vi "HEWH Draw Start GEA3 Commands.vi"(5 "Draw Station":string, 7 "GEA3?":bool, 8 "error in (no error)":errorcluster, 9 "Draw Parameters Seq":T1 {"Station D"."Time" format="%<%H:%M:%S>t"; "Station C"."Time" format="%<%H:%M:%S>t"; "Station B"."Time" format="%<%H:%M:%S>t"; "Station A"."Time" format="%<%H:%M:%S>t"}, 11 "GEA3 Reference Out":refnum<k24>) -> (0 "error out":errorcluster, 3 "GEA2 Reference Out":refnum<k24>)   [LabVIEW 2019]
uses:
  Type Definitions/HEWH Draw Parameters.ctl
  Type Definitions/PRAT Test.ctl
  Utility/Save File/File Setup (Public)/Type Definition/Save File HEWH Heating Control Mode.ctl
  Draw Water Specific/Type Definitions/Terminate Draw Conditions.ctl
  Type Definitions/HEWH Start Conditions.ctl
  Draw Water Specific/Type Definitions/Check Special Condtions.ctl
  Draw Water Specific/Type Definitions/HEWH Special Condition Check.ctl
  Type Definitions/HEWH Draw Flag ENUM.ctl
  C:/TechnologyLab/NI-2010/Drivers/GEA3 Toolkit/GEA3 DLL Source/GeaCommunication.dll
  Drivers/GEA3 Toolkit/GEA3 DLL Source/GeaCommunication.dll
  Drivers/GEA3 Toolkit/LabVIEW GEA3 Rev2 API Toolkit LV2016/type defs/ERD Write Data In.ctl
  Drivers/GEA3 Toolkit/LabVIEW GEA3 Rev2 API Toolkit LV2016/type defs/Data Type.ctl
  Utility/Save File/File Setup.lvlib
  Drivers/GEA3 Toolkit/LabVIEW GEA3 Rev2 API Toolkit LV2016/library/GEA2_Toolkit.lvlib
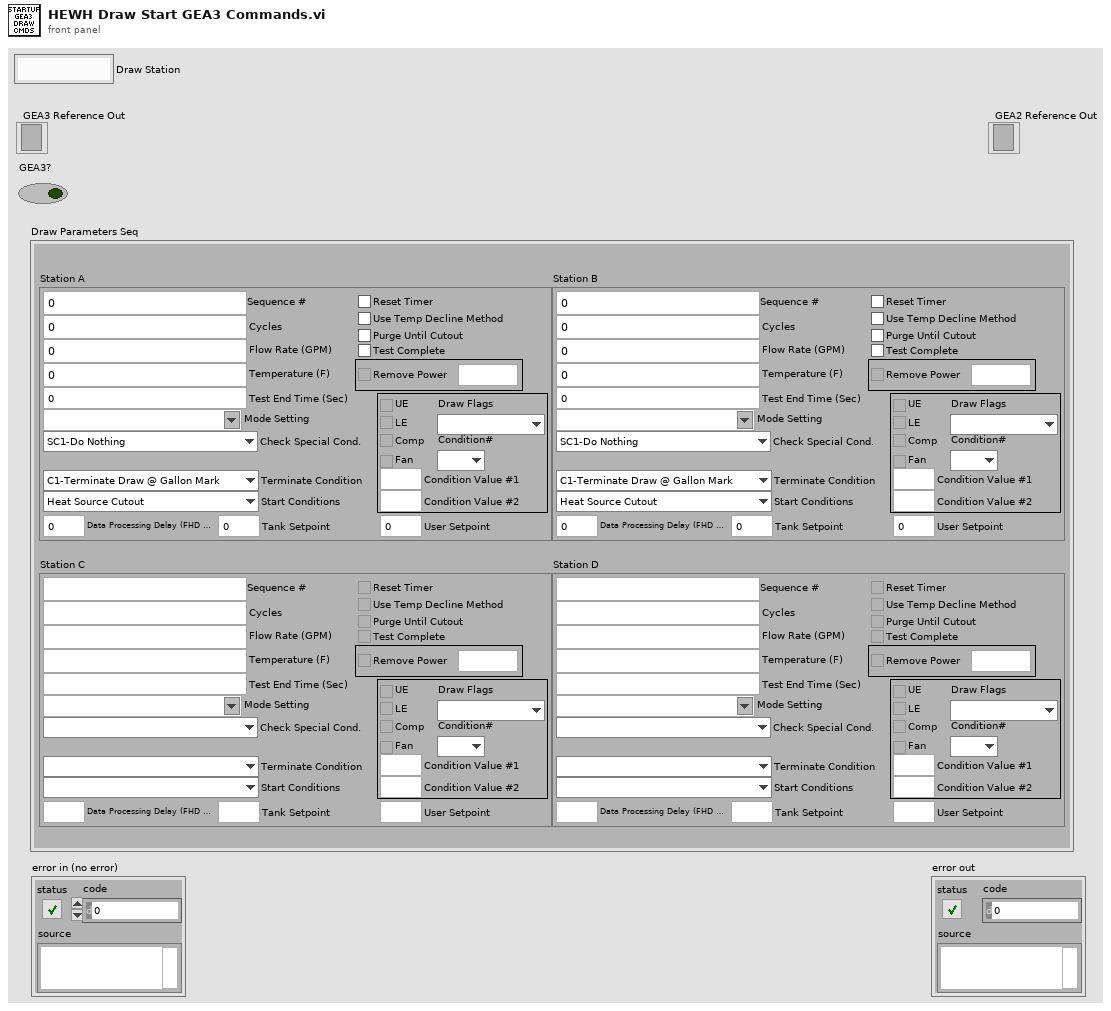
[diagram p1: front panel]
types:
  T1 = typedef "HEWH Draw Parameters.ctl" = cluster{"Draws Left":i32, "Draws Left Array":i32[], "Remaining Draws (A)":i32, "Remaining Draws (B)":i32, "Remaining Draws (C)":i32, "Remaining Draws (D)":i32, "Index of Element (A-D)":i32[], "Station A":T2, "Station B":T2, "Station C":T2, "Station D":T2}
  T2 = typedef "PRAT Test.ctl" = cluster{"Sequence #":dbl, "Cycles":i32, "Mode Setting":T3, "Flow Rate (GPM)":dbl, "Temperature (F)":dbl, "Reset Timer":bool, "Use Temp Decline Method":bool, "Terminate Condition":T4, "Condition Value #1":dbl, "UE":bool, "LE":bool, "Comp":bool, "Fan":bool, "Test End Time (Sec)":dbl, "Purge Until Cutout":bool, "Start Conditions":T5, "Condition Value #2":dbl, "Remove Power":bool, "Time":dbl, "Check Special Cond.":T6, "Condition#":T7, "Draw Flags":T8, "Data Processing Delay (FHD 15sec, UEF 5 Sec)":dbl, "Test Complete":bool, "User Setpoint":dbl, "Tank Setpoint":dbl}
  T3 = typedef "File Setup.lvlib/Save File HEWH Heating Control Mode.ctl" = string
  T4 = typedef "Terminate Draw Conditions.ctl" = enum16{"C1-Terminate Draw @ Gallon Mark", "C2-Special Last Draw (HU Test)", "C3-RTD Out <=", "C4-Mean Tank Temp <=", "C5-Decrease RTD Out (Deg F)", "C6-Time (Seconds)", "C7-Until Any Heat Source", "C8-Specific Heat Source", "C9-Do Nothing", "C10-Inlet Outlet RTD Temp Delta"}
  T5 = typedef "HEWH Start Conditions.ctl" = enum16{"Heat Source Cutout", "At Time (Seconds)", "Every X (Seconds)", "T2 >= X° Below Setpoint", "Seconds From Complete", "Wait for LE & Comp Cutout", "Wait for Comp Cutout", "Wait for LE Cutout", "Wait for UE Cutout", "Start Immediately"}
  T6 = typedef "Check Special Condtions.ctl" = enum16{"SC1-Do Nothing", "SC2-Check Heat Source (On-C2/Off-C1)", "SC3-Check Skip Condition", "SC4-Check Heat Source ON/Fail", "SC5-Keep Draw Valves Open", "SC6-Skip Purge"}
  T7 = typedef "HEWH Special Condition Check.ctl" = enum16{"N/A", "C1", "C2", "Reset/Fail", "Skip Draw Sequence"}
  T8 = typedef "HEWH Draw Flag ENUM.ctl" = enum16{"N/A", "None(0)", "Sml(1)", "Med(2)", "SmlMed(3)", "Lrg(4)", "SmlLrg(5)", "MedLrg(6)", "SmlMedLrg(7)"}
  T9 = typedef "GEA2_Toolkit.lvlib/ERD Write Data In.ctl" = cluster{"ERD Number":u16, "Data Type":T10, "Data":string}
  T10 = typedef "GEA2_Toolkit.lvlib/Data Type.ctl" = enum16{"string", "boolean", "uint8_t", "uint16_t", "uint32_t", "uint64_t", "int8_t", "int16_t", "int32_t", "int64_t"}
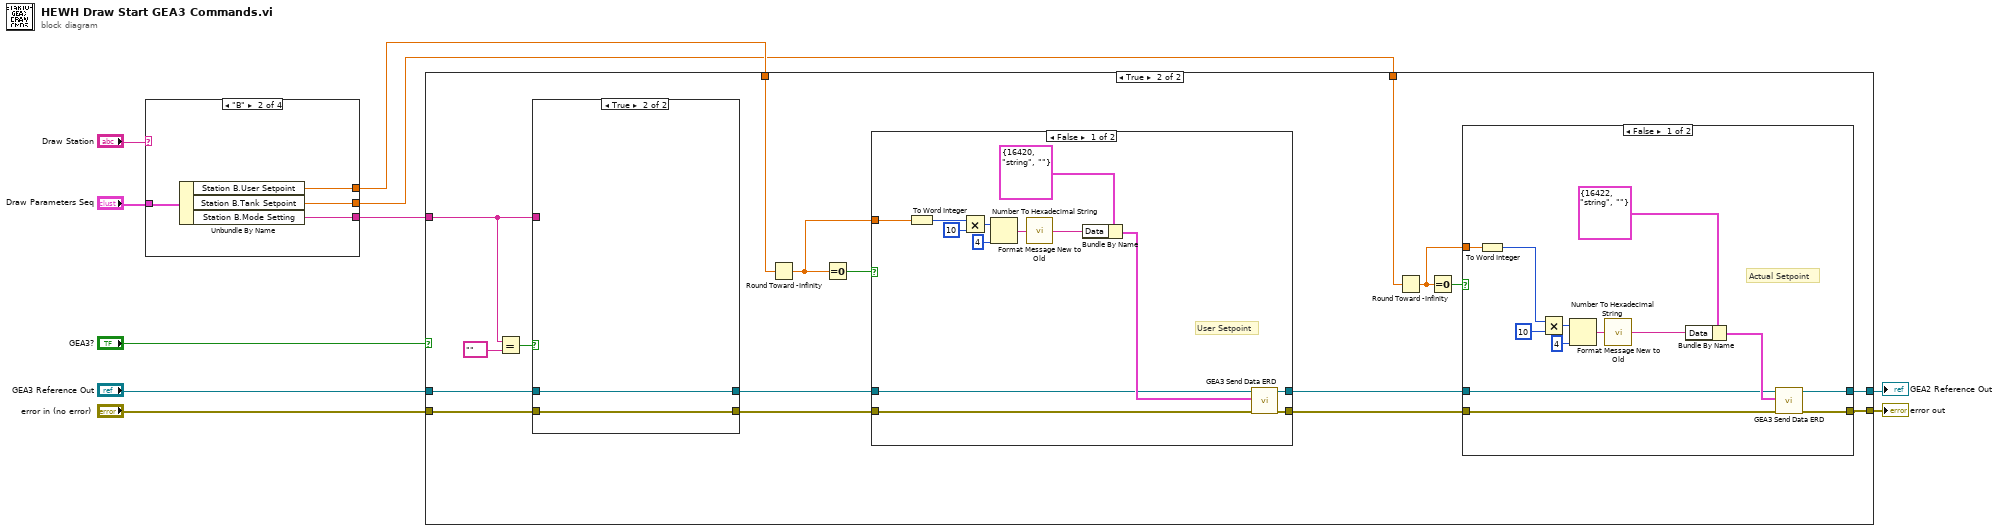
[diagram p0: block diagram]
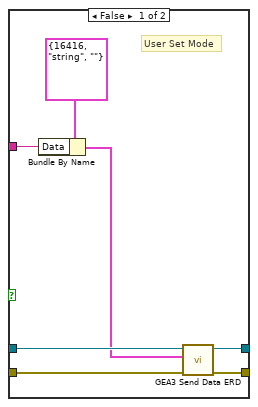
[diagram p5: hidden frame]
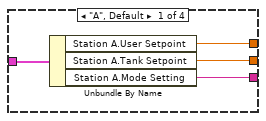
[diagram p6: hidden frame]
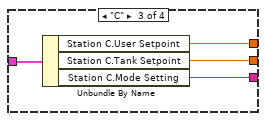
[diagram p7: hidden frame]
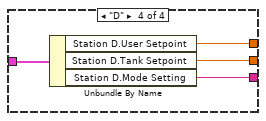
[diagram p8: hidden frame]
diagram:
  n1 = case shown="\"B\"" "Draw Station" {
    tunnel: "Draw Parameters Seq" -> [w14 w18 w22 w26]
    tunnel: [w13 w17 w21 w25] -> w7
    tunnel: [w12 w16 w20 w24] -> w5
    tunnel: [w11 w15 w19 w23] -> w4
    frame "A", Default {
      n2 = Unbundle By Name(w14) -> ("Station A.User Setpoint"=w12:dbl, "Station A.Tank Setpoint"=w11:dbl, "Station A.Mode Setting"=w13:T3)
    }
    frame "B" {
      n3 = Unbundle By Name(w18) -> ("Station B.User Setpoint"=w16:dbl, "Station B.Tank Setpoint"=w15:dbl, "Station B.Mode Setting"=w17:T3)
    }
    frame "C" {
      n4 = Unbundle By Name(w22) -> ("Station C.User Setpoint"=w20:dbl, "Station C.Tank Setpoint"=w19:dbl, "Station C.Mode Setting"=w21:T3)
    }
    frame "D" {
      n5 = Unbundle By Name(w26) -> ("Station D.User Setpoint"=w24:dbl, "Station D.Tank Setpoint"=w23:dbl, "Station D.Mode Setting"=w25:T3)
    }
  }
  n6 = case shown="True" "GEA3?" {
    tunnel: "GEA3 Reference Out" -> [w28 w45]
    tunnel: "error in (no error)" -> [w27 w44]
    tunnel: w7 -> [_ w31]
    tunnel: w5 -> [_ w42]
    tunnel: w4 -> [_ w39]
    tunnel: [w28 w35] -> w3
    tunnel: [w27 w34] -> w2
    frame False {
    }
    frame True {
      n7 = Equal?(x=w31, y=T3 "") -> (x = y?=w32:bool)
      n8 = case shown="True" w32 {
        tunnel: w44 -> [w82 w84]
        tunnel: [w81 w84] -> w29
        tunnel: w45 -> [w80 w83]
        tunnel: w31 -> [w77 _]
        tunnel: [w76 w83] -> w30
        frame False {
          # "User Set Mode"
          n9 = Bundle By Name(cluster=T9 {"ERD Number"=16416, "Data Type"=enum."string", "Data"=""} ("ERD Write Data In"), "Data"=w77) -> (w78:T9)
          n10 = call "GEA3 Send Data ERD.vi"("error in (no error)"=w82, "ERD Write Data In"=w78, ".NET Refnum in"=w80) -> ("error out"=w81:errorcluster, "GEA2 Reference Out"=w76:refnum<k24>)  [unwired: 5 in, 2 out]
        }
        frame True {
        }
      }
      n11 = Round Toward -Infinity(1:w42) -> (0:w41:dbl)
      n12 = Equal To 0?(x=w41) -> (x = 0?=w43:bool)
      n13 = case shown="False" w43 {
        tunnel: w29 -> [w63 w74]
        tunnel: w30 -> [w64 w75]
        tunnel: w41 -> [w66 _]
        tunnel: [w62 w75] -> w38
        tunnel: [w61 w74] -> w37
        frame False {
          # "User Setpoint"
          n14 = To Word Integer(number=w66) -> (16bit integer=w65:i16)
          n15 = Multiply(x=w65, y=i16 10) -> (x*y=w70:i16)
          n16 = Number To Hexadecimal String(1:i16 4 ("width (-)"), 2:w70) -> (0:w72:string)
          n17 = call "Format Message New to Old.vi"("Raw Message In"=w72) -> ("Conv Message Out"=w73:string)  [unwired: 14 in]
          n18 = Bundle By Name(cluster=T9 {"ERD Number"=16420, "Data Type"=enum."string", "Data"=""} ("ERD Write Data In"), "Data"=w73) -> (w67:T9)
          n19 = call "GEA3 Send Data ERD.vi"("error in (no error)"=w63, "ERD Write Data In"=w67, ".NET Refnum in"=w64) -> ("error out"=w61:errorcluster, "GEA2 Reference Out"=w62:refnum<k24>)  [unwired: 5 in, 2 out]
        }
        frame True {
        }
      }
      n20 = Round Toward -Infinity(1:w39) -> (0:w36:dbl)
      n21 = Equal To 0?(x=w36) -> (x = 0?=w40:bool)
      n22 = case shown="False" w40 {
        tunnel: w38 -> [w50 w60]
        tunnel: w37 -> [w51 w59]
        tunnel: [w49 w60] -> w35
        tunnel: [w48 w59] -> w34
        tunnel: w36 -> [w47 _]
        frame False {
          # "Actual Setpoint"
          n23 = To Word Integer(number=w47) -> (16bit integer=w46:i16)
          n24 = Multiply(x=w46, y=i16 10) -> (x*y=w55:i16)
          n25 = Number To Hexadecimal String(1:i16 4 ("width (-)"), 2:w55) -> (0:w57:string)
          n26 = call "Format Message New to Old.vi"("Raw Message In"=w57) -> ("Conv Message Out"=w58:string)  [unwired: 14 in]
          n27 = Bundle By Name(cluster=T9 {"ERD Number"=16422, "Data Type"=enum."string", "Data"=""} ("ERD Write Data In"), "Data"=w58) -> (w52:T9)
          n28 = call "GEA3 Send Data ERD.vi"("error in (no error)"=w51, "ERD Write Data In"=w52, ".NET Refnum in"=w50) -> ("error out"=w48:errorcluster, "GEA2 Reference Out"=w49:refnum<k24>)  [unwired: 5 in, 2 out]
        }
        frame True {
        }
      }
    }
  }
  "error out" <- w2
  "GEA2 Reference Out" <- w3
